vi "Abort.vi"(8 "error in (no error)":errorcluster, 11 "Sequence in":refnum<class "Sequence.lvclass">) -> (0 "error out":errorcluster, 3 "Sequence out":refnum<class "Sequence.lvclass">)   [LabVIEW 2020, in "VolatusSeq.lvlib" / "Sequence.lvclass"]
uses:
  Sequence.lvclass
  Sequence.lvclass/Sequence.ctl
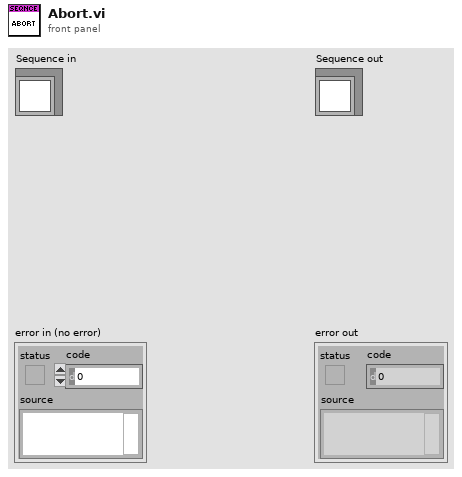
[diagram p1: front panel]
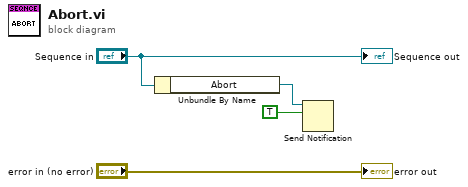
[diagram p0: block diagram]
diagram:
  n1 = Unbundle By Name("Sequence in") -> ("Abort"=w2:refnum<notifier>)
  n2 = Send Notification(notification=TRUE, notifier=w2) -> ()  [unwired: 1 in, 2 out]
  "error out" <- "error in (no error)"
  "Sequence out" <- "Sequence in"
